vi "PRIVATE.i attribute.vi"(0 "VI Refnum":refnum<vi>, 2 "CLASS.i attribute":T1, 3 "Action":T2(ring), 5 "error in (no error)":errorcluster) -> (14 "VI Refnum out":refnum<vi>, 16 "CLASS.i attribute out":T1, 19 "error out":errorcluster)   [LabVIEW 2014, in "CleanHandler.lvlib"]
doc: "This is a so-called functional global variable. It manages the access to a global variable in a thread-safe way. \n\nHere the attribute data of all instances of THIS class are stored. This is done for performance reasons.\n\nLicense Agreement for this software:\n\nCopyright (C)\nGesellschaft für Schwerionenforschung, GSI\nPlanckstr. 1\n64291 Darmstadt\nGermany\n\nContact: D.Beck@gsi.de \n\nThis program is free software; you can redistribute it and/or modify it under the terms of the GNU General Public License as published by the Free Software Foundation; either version 2 of the license, or (at your option) any later version.\n\nThis program is distributed in the hope that it will be useful, but WITHOUT ANY WARRANTY; without even the implied warranty of MERCHANTABILITY or FITNESS FOR A PARTICULAR PURPOSE. See the GNU General License for more details (http://www.gnu.org).\n\nGesellschaft für Schwerionenforschung, GSI\nPlanckstr. 1, 64291 Darmstadt, Germany\nFor all questions and ideas contact: M.Richter@gsi.de, H.Brand@gsi.de or D.Beck@gsi.de.\nLast update: 17-JUN-2004"
uses:
  CleanHandler.lvlib
  PRIVATE.i attribute.ctl
  CS_Core/CSSystem/CoreDefs/CoreDefs.error_type.ctl
  CS_Core/CSSystem/CoreLib/CoreLib.lvlib
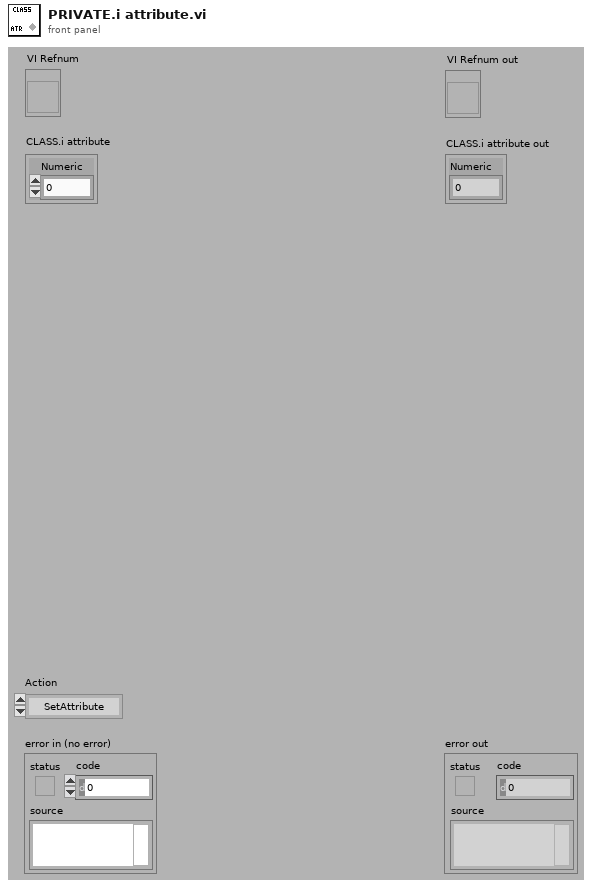
[diagram p1: front panel]
types:
  T1 = typedef "CleanHandler.lvlib/PRIVATE.i attribute.ctl" = cluster{"Numeric":dbl}
  T2 = enum16{"SetAttribute", "GetAttribute", "CreateAttribute", "DestroyAttribute", "DestroyAllAtributes"}
  T3 = typedef "CoreDefs.error_type.ctl" = enum16{"no error", "can't load process", "can't unload process", "process does not exist", "can't install process", "can't remove process", "unknown function", "time out", "can't execute function", "duplicate queue name", "super not found", "caller queue invalid", "can't ping process", "unknown error", "VISA Error", "VISA timeout", "GPIB timeout", "GPIB error", "communication error", "data type mismatch", "can't read data from OPC server", "can't write data to OPC server", "OET error", "function not implemented", "process already exists", "invalid Shared Variable name", "error writing Shared Variable", "error reading Shared Variable", "invalid client name", "corrupt database", "unknown class", "call not authorized", "parameter out of range", "OET timeout: can't get data to modify", "invalid queue name", "requested operation incompatible with current state", "event undefined", "event disabled", "state undefined", "caller is not a friend", "EventBuilder: bad eventID", "EventBuilder: no DAQ devices", "a thread must not stop itself", "UNUSED ELEMENT4", "DiscArchiver: eventData incomplete", "DiscArchiver: eventData does not belong to run", "DiscArchiver: can't open file", "DiscArchiver: can't write to file", "DiscArchiver: available disc space low", "can't acquire semaphore", "error reading data from database", "notifier object is not existing", "can't register process", "can't unregister process", "illegal event type", "object disabled", "object already exists", "can't change state", "Instrument not found", "no connection to remote node", "invalid reference", "N/A", "UNUSED ELEMENT 1", "element not found", "illegal TCP/IP connection detected", "object does not exist", "invalid access ID", "unknown CS system", "invalid privilige", "unsupported data type", "unsupported server type", "IO server already exists", "Shared Variable already exists"}
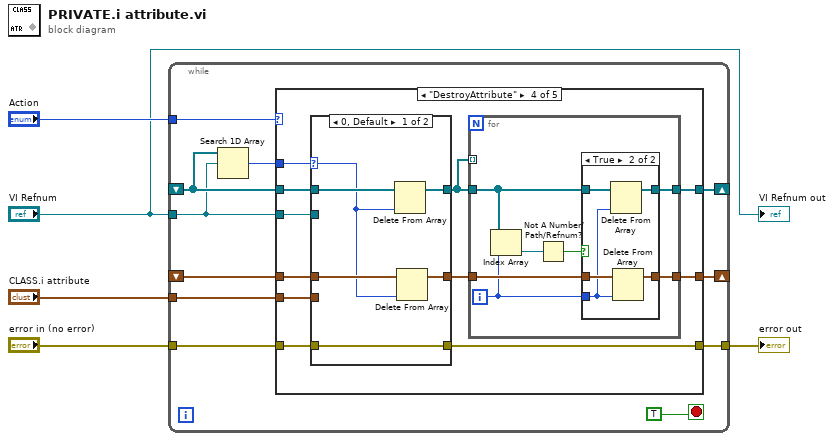
[diagram p0: block diagram]
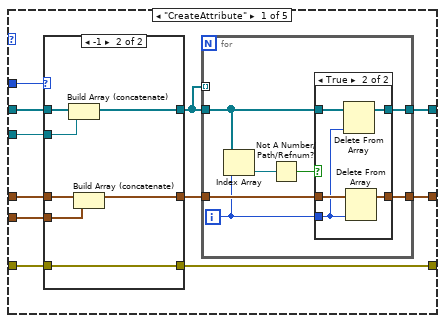
[diagram p2: hidden frame]
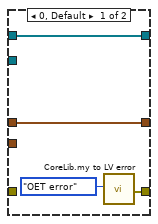
[diagram p4: hidden frame]
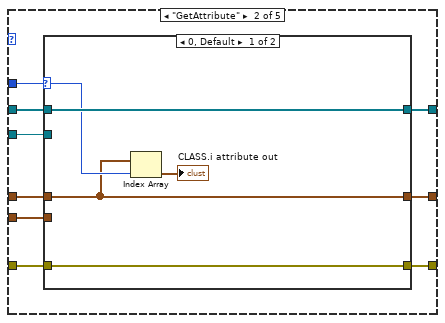
[diagram p5: hidden frame]
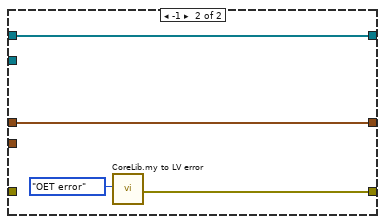
[diagram p6: hidden frame]
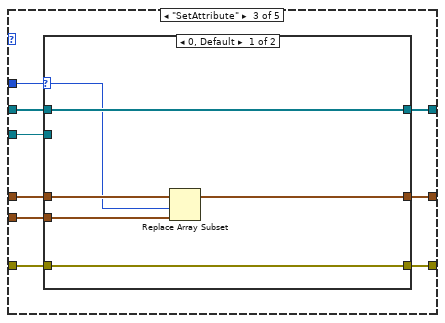
[diagram p7: hidden frame]
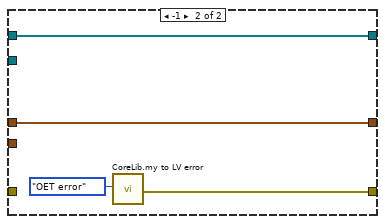
[diagram p8: hidden frame]
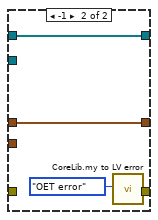
[diagram p10: hidden frame]
diagram:
  n1 = while {
    shift-right: [w10] -> _
    shift-left: _ -> [w11]
    tunnel: "Action" -> [w15]
    shift-right: [w12] -> _
    shift-left: _ -> [w8]
    tunnel: "VI Refnum" -> [w7]
    tunnel: "error in (no error)" -> [w14]
    tunnel: [w13] -> w3
    tunnel: "CLASS.i attribute" -> [w9]
    stop <- TRUE stop-if-true
    n2 = Search 1D Array(1D array=w8, element=w7) -> (index of element=w6:i32)  [unwired: 1 in]
    n3 = case shown="\"DestroyAttribute\"" w15 {
      tunnel: w8 -> [w25 w59 w77 w98 _]
      tunnel: w7 -> [w24 w57 w75 w97 _]
      tunnel: w14 -> [w27 w61 w79 w100 w125]
      tunnel: [w26 w60 w78 w99 w125] -> w13
      tunnel: [w20 w58 w76 w92 _] -> w12
      tunnel: w11 -> [w23 w56 w74 w96 _]
      tunnel: [w18 w55 w73 w91 _] -> w10
      tunnel: w9 -> [w22 w54 w72 w95 _]
      tunnel: w6 -> [w21 w53 w71 w94 _]
      frame "CreateAttribute" {
        n4 = case shown="-1" w21 {
          tunnel: w27 -> [_ w52]
          tunnel: [w44 w52] -> w26
          tunnel: w25 -> [w43 w51]
          tunnel: [w43 w50] -> w17
          tunnel: w24 -> [_ w49]
          tunnel: w23 -> [w42 w48]
          tunnel: [w42 w47] -> w19
          tunnel: w22 -> [_ w46]
          frame 0, Default {
            n5 = call "CoreLib.my to LV error.vi"("ErrorTypes"=CoreDefs.error_type."OET error") -> ("myErrorCluster"=w44:errorcluster)  [unwired: 17 in, 1 out]
          }
          frame -1 {
            n6 = Build Array (concatenate)(w51, w49) -> (w50:refnum<vi>[])
            n7 = Build Array (concatenate)(w48, w46) -> (w47:T1[])
          }
        }
        n8 = for {
          tunnel: w17 -> [w30]
          tunnel: [w29] -> w20
          tunnel: [w34] -> w18
          tunnel: w19 -> [w33]
          tunnel: w17 -> [_] mode=indexing
          i -> [w28]
          n9 = Index Array(array=w30, index=w28) -> (element=w31:refnum<vi>)
          n10 = Not A Number/Path/Refnum?(number/path/refnum=w31) -> (NaN/Path/Refnum?=w32:bool)
          n11 = case shown="True" w32 {
            tunnel: [w36 w41] -> w34
            tunnel: w33 -> [w36 w40]
            tunnel: [w35 w38] -> w29
            tunnel: w30 -> [w35 w39]
            tunnel: w28 -> [_ w37]
            frame False {
            }
            frame True {
              n12 = Delete From Array(array=w39, index=w37) -> (array with subset deleted=w38:refnum<vi>[])  [unwired: 1 in, 1 out]
              n13 = Delete From Array(array=w40, index=w37) -> (array with subset deleted=w41:T1[])  [unwired: 1 in, 1 out]
            }
          }
        }
      }
      frame "GetAttribute" {
        n14 = case shown="0, Default" w53 {
          selector: w53 -> [w64 _]
          tunnel: w61 -> [w66 _]
          tunnel: [w66 w69] -> w60
          tunnel: w59 -> [w65 w68]
          tunnel: [w65 w68] -> w58
          tunnel: w57 -> [_ _]
          tunnel: w56 -> [w63 w67]
          tunnel: [w63 w67] -> w55
          tunnel: w54 -> [_ _]
          frame 0, Default {
            n15 = Index Array(array=w63, index=w64) -> (element=→"CLASS.i attribute out":T1)
          }
          frame -1 {
            n16 = call "CoreLib.my to LV error.vi"("ErrorTypes"=CoreDefs.error_type."OET error") -> ("myErrorCluster"=w69:errorcluster)  [unwired: 17 in, 1 out]
          }
        }
      }
      frame "SetAttribute" {
        n17 = case shown="0, Default" w71 {
          selector: w71 -> [w81 _]
          tunnel: w79 -> [w85 _]
          tunnel: [w85 w88] -> w78
          tunnel: w77 -> [w84 w87]
          tunnel: [w84 w87] -> w76
          tunnel: w75 -> [_ _]
          tunnel: w74 -> [w83 w86]
          tunnel: [w82 w86] -> w73
          tunnel: w72 -> [w80 _]
          frame 0, Default {
            n18 = Replace Array Subset(array=w83, new element=w80, index=w81) -> (w82:T1[])
          }
          frame -1 {
            n19 = call "CoreLib.my to LV error.vi"("ErrorTypes"=CoreDefs.error_type."OET error") -> ("myErrorCluster"=w88:errorcluster)  [unwired: 17 in, 1 out]
          }
        }
      }
      frame "DestroyAttribute" {
        n20 = case shown="0, Default" w94 {
          selector: w94 -> [w116 _]
          tunnel: w100 -> [w120 _]
          tunnel: [w120 w123] -> w99
          tunnel: w98 -> [w119 w122]
          tunnel: [w118 w122] -> w90
          tunnel: w97 -> [_ _]
          tunnel: w96 -> [w117 w121]
          tunnel: [w115 w121] -> w93
          tunnel: w95 -> [_ _]
          frame 0, Default {
            n21 = Delete From Array(array=w119, index=w116) -> (array with subset deleted=w118:refnum<vi>[])  [unwired: 1 in, 1 out]
            n22 = Delete From Array(array=w117, index=w116) -> (array with subset deleted=w115:T1[])  [unwired: 1 in, 1 out]
          }
          frame -1 {
            n23 = call "CoreLib.my to LV error.vi"("ErrorTypes"=CoreDefs.error_type."OET error") -> ("myErrorCluster"=w123:errorcluster)  [unwired: 17 in, 1 out]
          }
        }
        n24 = for {
          tunnel: w90 -> [w103]
          tunnel: [w102] -> w92
          tunnel: [w107] -> w91
          tunnel: w93 -> [w106]
          tunnel: w90 -> [_] mode=indexing
          i -> [w101]
          n25 = Index Array(array=w103, index=w101) -> (element=w104:refnum<vi>)
          n26 = Not A Number/Path/Refnum?(number/path/refnum=w104) -> (NaN/Path/Refnum?=w105:bool)
          n27 = case shown="True" w105 {
            tunnel: [w109 w114] -> w107
            tunnel: w106 -> [w109 w113]
            tunnel: [w108 w111] -> w102
            tunnel: w103 -> [w108 w112]
            tunnel: w101 -> [_ w110]
            frame False {
            }
            frame True {
              n28 = Delete From Array(array=w112, index=w110) -> (array with subset deleted=w111:refnum<vi>[])  [unwired: 1 in, 1 out]
              n29 = Delete From Array(array=w113, index=w110) -> (array with subset deleted=w114:T1[])  [unwired: 1 in, 1 out]
            }
          }
        }
      }
      frame "DestroyAllAtributes" {
      }
    }
  }
  "error out" <- w3
  "VI Refnum out" <- "VI Refnum"
